vi "Get Timeout.vi"(8 "error in (no error)":errorcluster, 11 "JKI SM in":refnum<class "JKI SM.lvclass">) -> (0 "error out":errorcluster, 2 "Timeout (ms)":i32, 3 "JKI SM out":refnum<class "JKI SM.lvclass">)   [LabVIEW 2020, in "JKI State Machine API.lvlib" / "JKI SM.lvclass"]
uses:
  JKI SM.lvclass
  JKI SM.lvclass/JKI SM.ctl
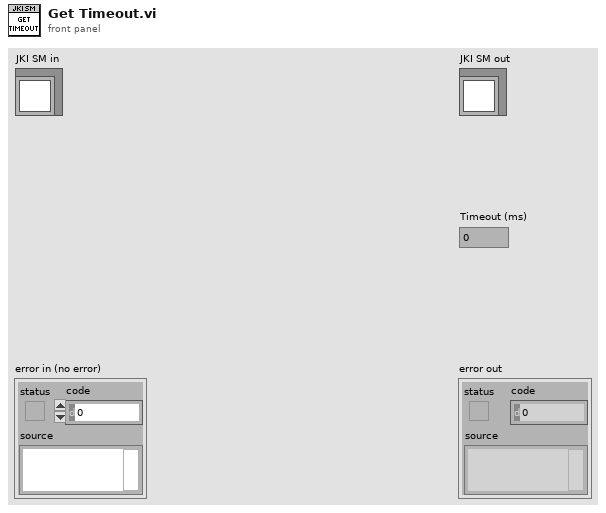
[diagram p1: front panel]
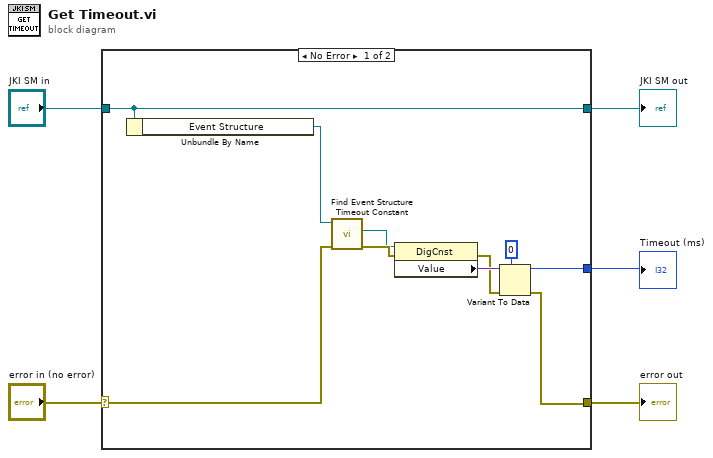
[diagram p0: block diagram]
diagram:
  n1 = case shown="No Error" "error in (no error)" {
    selector: "error in (no error)" -> [w13 w17]
    tunnel: [w7 w17] -> w4
    tunnel: [w15 w16] -> w2
    tunnel: "JKI SM in" -> [w15 w16]
    tunnel: [w9 _] -> w1
    frame No Error {
      n2 = Unbundle By Name(w15) -> ("Event Structure"=w14:refnum<vi>)
      n3 = call "Find Event Structure Timeout Constant.vi"("error in (no error)"=w13, "EventStructure in"=w14) -> ("error out"=w12:errorcluster, "DigitalNumericConstant out"=w6:refnum<vi>)  [unwired: 8 in]
      n4 = property class="DigCnst"(reference=w6, error in=w12) -> (error out=w8:errorcluster, "Value"=w10:variant)  [unwired: 1 out]
      n5 = Variant To Data(error in=w8, type=0 ("Numeric"), Variant=w10) -> (data=w9:i32, error out=w7:errorcluster)
    }
    frame Error {
    }
  }
  "error out" <- w4
  "JKI SM out" <- w2
  "Timeout (ms)" <- w1
